vi "set Lua keyword style.vi"(0 "ScintillaNET in":refnum<class "ScintillaNET.lvclass">, 5 "keyword group (1~7)":i32=1, 7 "keyword":string[](array[string]), 9 "Color style":T1, 11 "error in (no error)":errorcluster) -> (4 "ScintillaNET out":refnum<class "ScintillaNET.lvclass">, 15 "error out":errorcluster)   [LabVIEW 2018, in "ScintillaNET.lvclass"]
uses:
  ScintillaNET.lvclass
  style index Lua.ctl
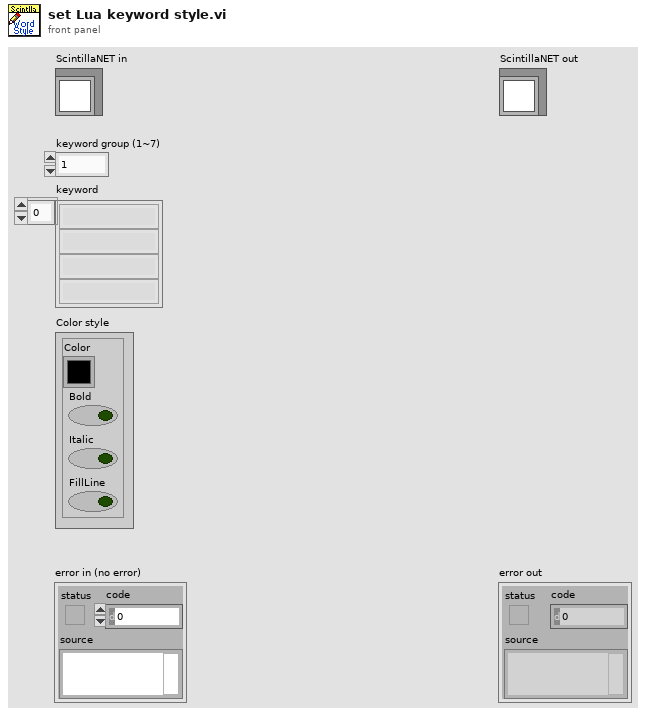
[diagram p1: front panel]
types:
  T1 = cluster{"Color":u32, "Bold":bool, "Italic":bool, "FillLine":bool}
  T2 = typedef "ScintillaNET.lvclass/style index Lua.ctl" = enum16{"Default", "Comment", "CommentLine", "CommentDoc", "Number", "Word", "String", "Character", "LiteralString", "Preprocessor", "Operator", "Identifier", "StringEol", "Word2", "Word3", "Word4", "Word5", "Word6", "Word7", "Word8", "Label"}
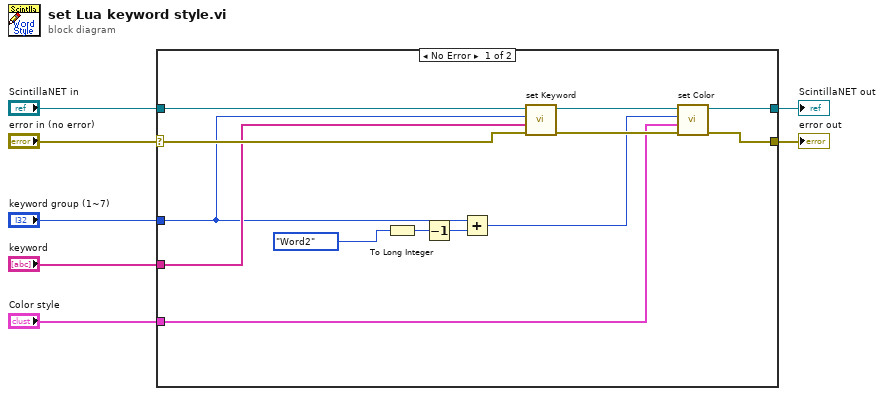
[diagram p0: block diagram]
diagram:
  n1 = case shown="No Error" "error in (no error)" {
    selector: "error in (no error)" -> [w16 w22]
    tunnel: [w15 w22] -> w6
    tunnel: [w17 w21] -> w4
    tunnel: "ScintillaNET in" -> [w18 w21]
    tunnel: "keyword" -> [w14 _]
    tunnel: "Color style" -> [w13 _]
    tunnel: "keyword group (1~7)" -> [w12 _]
    frame No Error {
      n2 = To Long Integer(number=style_index_Lua."Word2" ("style index Lua")) -> (32bit integer=w9:i32)
      n3 = Decrement(x=w9) -> (x-1=w8:i32)
      n4 = Add(x=w12, y=w8) -> (x+y=w10:i32)
      n5 = call "set Keyword.vi"("error in (no error)"=w16, "keyword"=w14, "keyword index"=w12, "ScintillaNET in"=w18) -> ("error out"=w19:errorcluster, "ScintillaNET out"=w20:refnum<class "ScintillaNET.lvclass">)  [unwired: 6 in]
      n6 = call "set Color.vi"("error in (no error)"=w19, "Color style"=w13, "style index"=w10, "ScintillaNET in"=w20) -> ("error out"=w15:errorcluster, "ScintillaNET out"=w17:refnum<class "ScintillaNET.lvclass">)  [unwired: 6 in]
    }
    frame Error {
    }
  }
  "error out" <- w6
  "ScintillaNET out" <- w4
